vi "Init Control.vi"(5 "Group":refnum<class "Group DBL.lvclass">, 6 "Period ms":i64, 7 "VolatusAPI":refnum<class "VolatusAPI.lvclass">, 8 "error in (no error)":errorcluster, 9 "Control MsgQ":refnum<class "MessageQ.lvclass">, 10 "Config Element":refnum<class "Config Element.lvclass">, 11 "Valve in":refnum<class "InterlockControl.lvclass">) -> (0 "error out":errorcluster, 3 "Valve out":refnum<class "InterlockControl.lvclass">)   [LabVIEW 2020, in "VolatusControl.lvlib" / "InterlockControl.lvclass"]
uses:
  InterlockControl.lvclass
  lv-cdm/CDM-Config/Config Element/Config Element.lvclass
  Volatus/VolatusAPI/VolatusAPI.lvclass
  Volatus/MessageQ/MessageQ.lvclass
  lv-vecto/Vecto/Group DBL/Group DBL.lvclass
  C:/dev/lv20CE/relink/lv-vecto/Vecto/Group/Group.lvclass
  Inhibit Logic.ctl
  Inhibit Condition.ctl
  Inhibit Comparison.ctl
  InterlockControl.lvclass/InterlockControl.ctl
  lv-cdm/CDM-Config/Config Element/Owner.vi
  lv-cdm/CDM-Config/Config Manager/Lookup Descendant.vi
  lv-vecto/Vecto/Group/Group.lvclass
  lv-cdm/CDM-Config/Config Filter/Config Lookup.lvclass
  lv-vecto/Vecto/Vecto.lvlib
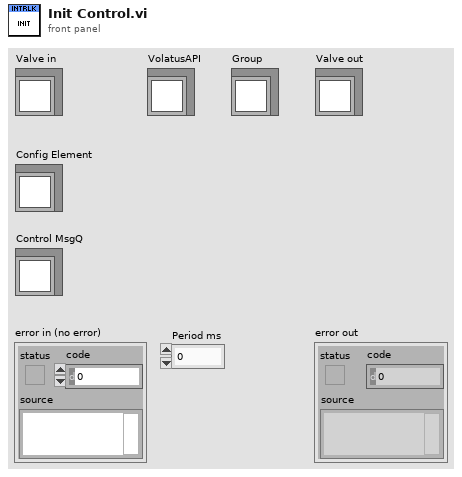
[diagram p1: front panel]
types:
  T1 = typedef "VolatusControl.lvlib/InterlockControl.lvclass/Inhibit Logic.ctl" = enum16{"Any", "All"}
  T2 = typedef "VolatusControl.lvlib/InterlockControl.lvclass/Inhibit Condition.ctl" = cluster{"Channel Name":string, "Comparison":T3, "Value":dbl}
  T3 = typedef "VolatusControl.lvlib/InterlockControl.lvclass/Inhibit Comparison.ctl" = enum16{"Equal", "Less Than", "Greater Than"}
  T4 = typedef "CDM-Config.lvlib/Value Type.ctl" = enum16{"String", "Number", "Bool", "Object", "Array"}
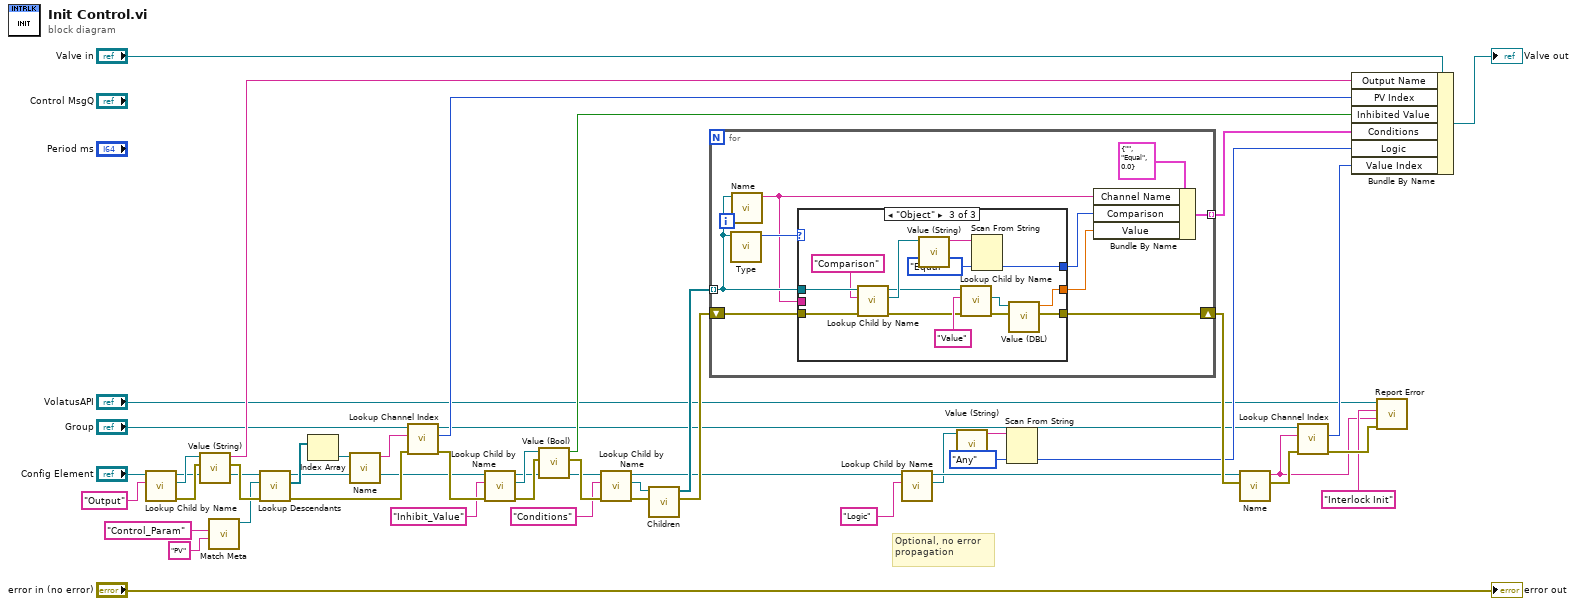
[diagram p0: block diagram]
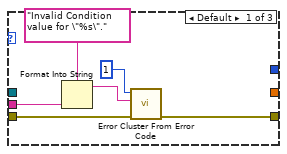
[diagram p2: hidden frame]
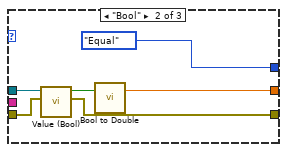
[diagram p3: hidden frame]
diagram:
  # "Optional, no error propagation"
  n1 = call "Lookup Child by Name.vi"("Name"="Output", "Config Element in"="Config Element") -> ("error out"=w45:errorcluster, "Child"=w39:refnum<class "Config Element.lvclass">, "Config Element out"=w34:refnum<class "Config Element.lvclass">)  [unwired: 6 in, 1 out]
  n2 = call "Value (String).vi"("error in (no error)"=w45, "Config Element in"=w39) -> ("error out"=w44:errorcluster, "String Value"=w37:string)  [unwired: 8 in]
  n3 = call "Match Meta.vi"("Value (Any)"="PV" ("Name"), "Name"="Control_Param") -> ("Config Lookup out"=w33:refnum<class "Config Lookup.lvclass">)  [unwired: 8 in, 1 out]
  n4 = call "Lookup Descendants.vi"("error in (no error)"=w44, "Lookup"=w33, "Config Element in"=w34) -> ("error out"=w31:errorcluster, "Descendants"=w32:refnum<class "Config Element.lvclass">[], "Config Element out"=w23:refnum<class "Config Element.lvclass">)  [unwired: 6 in]
  n5 = Index Array(array=w32) -> (element=w29:refnum<class "Config Element.lvclass">)  [unwired: 1 in]
  n6 = call "Name.vi"("Config Element in"=w29) -> ("Name"=w30:string)  [unwired: 9 in, 1 out]
  n7 = call "Lookup Channel Index.vi"("error in (no error)"=w31, "Channel Name"=w30, "Group in"="Group") -> ("error out"=w25:errorcluster, "Index"=w27:i32, "Group out"=w6:refnum<class "Group DBL.lvclass">)  [unwired: 6 in]
  n8 = call "Lookup Child by Name.vi"("error in (no error)"=w25, "Name"="Inhibit_Value", "Config Element in"=w23) -> ("error out"=w22:errorcluster, "Child"=w26:refnum<class "Config Element.lvclass">, "Config Element out"=w20:refnum<class "Config Element.lvclass">)  [unwired: 5 in, 1 out]
  n9 = call "Value (Bool).vi"("error in (no error)"=w22, "Config Element in"=w26) -> ("error out"=w46:errorcluster, "Bool Value"=w21:bool)  [unwired: 8 in]
  n10 = call "Lookup Child by Name.vi"("error in (no error)"=w46, "Name"="Conditions", "Config Element in"=w20) -> ("error out"=w18:errorcluster, "Child"=w17:refnum<class "Config Element.lvclass">, "Config Element out"=w12:refnum<class "Config Element.lvclass">)  [unwired: 5 in, 1 out]
  n11 = call "Children.vi"("error in (no error)"=w18, "Config Element in"=w17) -> ("error out"=w16:errorcluster, "Elements"=w15:refnum<class "Config Element.lvclass">[])  [unwired: 8 in]
  n12 = for {
    shift-right: [w55] -> w47
    shift-left: w16 -> [w56]
    tunnel: w15 -> [w54] mode=indexing
    tunnel: [w49] -> w14 mode=indexing
    n13 = call "Type.vi"("Config Element in"=w54) -> ("Value Type"=w57:T4)  [unwired: 9 in, 1 out]
    n14 = call "Name.vi"("Config Element in"=w54) -> ("Name"=w52:string)  [unwired: 9 in, 1 out]
    n15 = case shown="\"Object\"" w57 {
      tunnel: w54 -> [_ w69 w83]
      tunnel: w56 -> [w63 w68 w82]
      tunnel: [w62 w67 w71] -> w55
      tunnel: w52 -> [w60 _ _]
      tunnel: [_ w65 w70] -> w51
      tunnel: [_ Inhibit_Comparison."Equal" ("Comparison") w80] -> w50
      frame Default {
        n16 = Format Into String(format string="Invalid Condition value for \"%s\".", w60) -> (resulting string=w58:string)  [unwired: 2 in, 1 out]
        n17 = call <vilib>:"Error Cluster From Error Code.vi"("error in (no error)"=w63, "error message (\"\")"=w58, "error code (0)"=1) -> ("error out"=w62:errorcluster)  [unwired: 6 in]
      }
      frame "Bool" {
        n18 = call "Value (Bool).vi"("error in (no error)"=w68, "Config Element in"=w69) -> ("error out"=w67:errorcluster, "Bool Value"=w66:bool)  [unwired: 8 in]
        n19 = call "Bool to Double.vi"("Bool"=w66) -> ("Double"=w65:dbl)  [unwired: 2 in]
      }
      frame "Object" {
        n20 = call "Lookup Child by Name.vi"("error in (no error)"=w82, "Name"="Comparison", "Config Element in"=w83) -> ("error out"=w74:errorcluster, "Child"=w77:refnum<class "Config Element.lvclass">, "Config Element out"=w75:refnum<class "Config Element.lvclass">)  [unwired: 5 in, 1 out]
        n21 = call "Value (String).vi"("Config Element in"=w77) -> ("String Value"=w78:string)  [unwired: 9 in, 1 out]
        n22 = call "Lookup Child by Name.vi"("error in (no error)"=w74, "Name"="Value", "Config Element in"=w75) -> ("error out"=w73:errorcluster, "Child"=w72:refnum<class "Config Element.lvclass">)  [unwired: 5 in, 2 out]
        n23 = Scan From String(input string=w78, default 1=Inhibit_Comparison."Equal" ("Comparison")) -> (output 1=w80:T3)  [unwired: 3 in, 3 out]
        n24 = call "Value (DBL).vi"("error in (no error)"=w73, "Config Element in"=w72) -> ("error out"=w71:errorcluster, "DBL Value"=w70:dbl)  [unwired: 8 in]
      }
    }
    n25 = Bundle By Name(cluster=T2 {"Channel Name"="", "Comparison"=enum."Equal", "Value"=0.0} ("Inhibit Input"), "Channel Name"=w52, "Comparison"=w50, "Value"=w51) -> (w49:T2)
  }
  n26 = call "Lookup Child by Name.vi"("Name"="Logic", "Config Element in"=w12) -> ("Child"=w10:refnum<class "Config Element.lvclass">, "Config Element out"=w11:refnum<class "Config Element.lvclass">)  [unwired: 6 in, 2 out]
  n27 = call "Value (String).vi"("Config Element in"=w10) -> ("String Value"=w9:string)  [unwired: 9 in, 1 out]
  n28 = Scan From String(input string=w9, default 1=Inhibit_Logic."Any" ("Logic")) -> (output 1=w7:T1)  [unwired: 3 in, 3 out]
  n29 = call "Name.vi"("error in (no error)"=w47, "Config Element in"=w11) -> ("error out"=w4:errorcluster, "Name"=w1:string)  [unwired: 8 in]
  n30 = call "Lookup Channel Index.vi"("error in (no error)"=w4, "Channel Name"=w1, "Group in"=w6) -> ("error out"=w48:errorcluster, "Index"=w5:i32)  [unwired: 6 in, 1 out]
  n31 = Bundle By Name(cluster="Valve in", "Output Name"=w37, "PV Index"=w27, "Inhibited Value"=w21, "Conditions"=w14, "Logic"=w7, "Value Index"=w5) -> (→"Valve out":refnum<class "InterlockControl.lvclass">)
  n32 = call "Report Error.vi"("error in (no error)"=w48, "Message"=w1, "Context"="Interlock Init", "VolatusAPI in"="VolatusAPI") -> ()  [unwired: 6 in, 2 out]
  "error out" <- "error in (no error)"
